vi "Asteroid_checkInRange.vi"(1 "AsteroidData":T2={"Veloc"=0.0, "Direction"=0.0, "Size"=0, "displayRef"=refnum, "Max X"=0.0, "Max Y"=0.0, "Xpos"=0.0, "Ypos"=0.0, "ID"=0, "Config"={"SpaceShip"={"Angle"=30.0, "SideLenght"=2.0, "MaxLinearVeloc"=10.0, "MaxAngularVeloc"=10.0, "LinearAceleration"=1.0, "AngularAceleration"=1.0}, "Physics"={"LinearDragFactor"=1.0, "AngularDragFactor"=1.0}, "Asteroids"={"MaxSize"=6.0, "MaxDivisions"=3, "MaxVeloc"=8.0, "MinVeloc"=1.0, "Fill"=FALSE}, "Environment"={"MaxAsteroids"=10, "TimeIncrement"=0.1, "AsterProbCreation"=0.1}, "Shots"={"MinTimeShots"=10.0, "ShotSize"=0.1, "ShotSpeed"=0.1}}}) -> (0 "NextState":T1)   [LabVIEW 2017]
uses:
  Asteroid_data.ctl
  GameConfig/GameConfig_data.ctl
  Asteroid_states.ctl
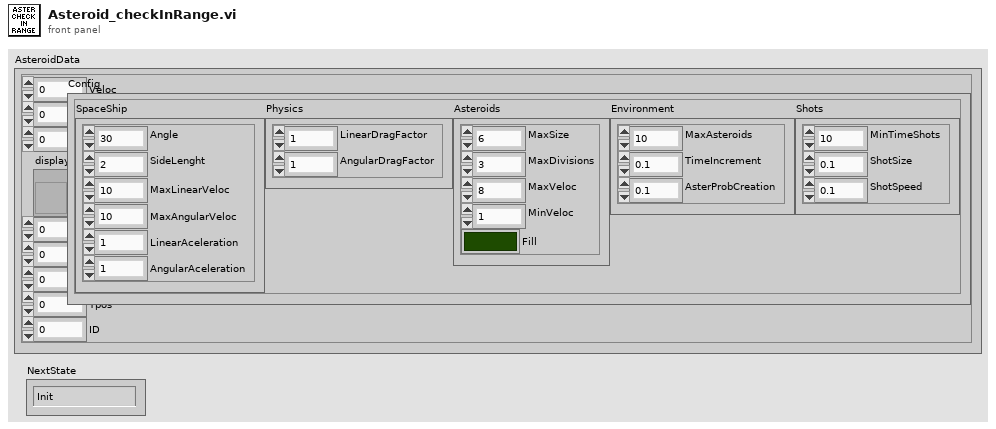
[diagram p1: front panel]
types:
  T1 = typedef "Asteroid_states.ctl" = enum16{"Init", "Move", "Split", "Draw", "Destroy"}
  T2 = typedef "Asteroid_data.ctl" = cluster{"Veloc":dbl, "Direction":dbl, "Size":i32, "displayRef":refnum<vi>, "Max X":dbl, "Max Y":dbl, "Xpos":dbl, "Ypos":dbl, "ID":i32, "Config":T3}
  T3 = typedef "GameConfig_data.ctl" = cluster{"SpaceShip":cluster{"Angle":dbl, "SideLenght":dbl, "MaxLinearVeloc":dbl, "MaxAngularVeloc":dbl, "LinearAceleration":dbl, "AngularAceleration":dbl}, "Physics":cluster{"LinearDragFactor":dbl, "AngularDragFactor":dbl}, "Asteroids":cluster{"MaxSize":dbl, "MaxDivisions":i32, "MaxVeloc":dbl, "MinVeloc":dbl, "Fill":bool}, "Environment":cluster{"MaxAsteroids":i32, "TimeIncrement":dbl, "AsterProbCreation":dbl}, "Shots":cluster{"MinTimeShots":dbl, "ShotSize":dbl, "ShotSpeed":dbl}}
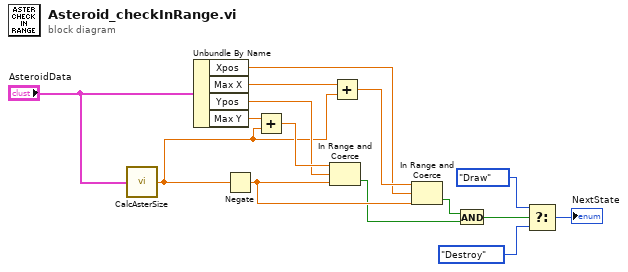
[diagram p0: block diagram]
diagram:
  n1 = call "CalcAsterSize.vi"("AsteroidData"="AsteroidData") -> ("AsteroidSize"=w10:dbl)
  n2 = Unbundle By Name("AsteroidData") -> ("Xpos"=w7:dbl, "Max X"=w11:dbl, "Ypos"=w12:dbl, "Max Y"=w14:dbl)
  n3 = Negate(x=w10) -> (-x=w8:dbl)
  n4 = Add(x=w14, y=w10) -> (x+y=w13:dbl)
  n5 = In Range and Coerce(upper limit=w13, x=w12, lower limit=w8) -> (In Range?=w5:bool)  [unwired: 1 out]
  n6 = Add(x=w11, y=w10) -> (x+y=w9:dbl)
  n7 = In Range and Coerce(upper limit=w9, x=w7, lower limit=w8) -> (In Range?=w6:bool)  [unwired: 1 out]
  n8 = And(x=w6, y=w5) -> (x .and. y?=w4:bool)
  n9 = Select(t=Asteroid_states."Draw" ("Asteroid_states"), s=w4, f=Asteroid_states."Destroy" ("Asteroid_states")) -> (s? t:f=→"NextState":T1)
